vi "Actor Core.vi"(8 "error in":errorcluster, 11 "XBoxController in":refnum<class "XBoxController.lvclass">) -> (0 "error out":errorcluster, 3 "Actor out":refnum<class "Actor.lvclass">)   [LabVIEW 2013, in "XBoxController.lvlib" / "XBoxController.lvclass"]
doc: "(<B>Filename</B>: Actor Framework.lvlib:Actor.lvclass:Actor Core.vi)\n\nReceives messages to the actor, reacts to them, and initiates any error handling that may shut the actor down.\n\nDescendant classes may override this VI to append parallel tasks for the actor to complete while it handles messages. Overrides use the Call Parent Method node."
uses:
  XBoxController.lvclass
  <vilib>/ActorFramework/Actor/Actor.lvclass
  XBoxController.lvclass/XBoxController.ctl
panel:
  in  "Tab Control":enum32{"Joysticks", "Page 2"}(tab)
  in  "XboxJoysticks":T1 {"RightJoystick"."Right" scale=-1.0..1.0; "RightJoystick"."Forward" scale=-1.0..1.0; "LeftJoystick"."Right" scale=-1.0..1.0; "LeftJoystick"."Forward" scale=-1.0..1.0}
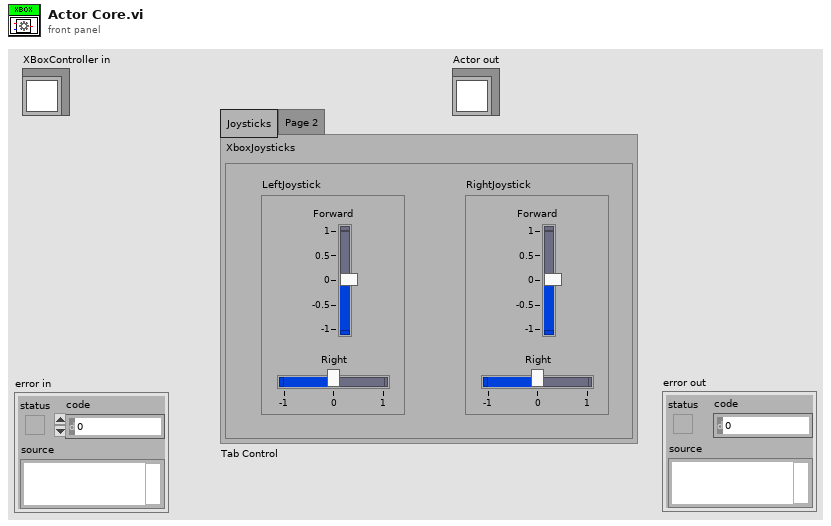
[diagram p1: front panel]
types:
  T1 = cluster{"LeftJoystick":cluster{"Forward":dbl, "Right":dbl}, "RightJoystick":cluster{"Forward":dbl, "Right":dbl}}
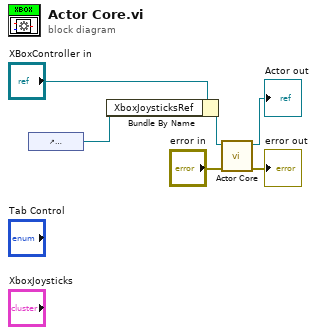
[diagram p0: block diagram]
diagram:
  n1 = control-ref of="XboxJoysticks"() -> (w1:refnum<vi>)
  n2 = Bundle By Name(cluster="XBoxController in", "XboxJoysticksRef"=w1) -> (w2:refnum<class "XBoxController.lvclass">)
  n3 = call-parent "Actor Core.vi"("error in"="error in", "Actor in"=w2) -> ("error out"=→"error out":errorcluster, "Actor out"=→"Actor out":refnum<class "Actor.lvclass">)  [unwired: 8 in]
